vi "Configure Protocol Settings.vi"(8 "error in":errorcluster, 11 "Protocol settings":T1={"Protocol capture resource name"="", "Data line"=0, "Channel"=0, "Clock rate"=12288000, "Number of words"=19200, "Sensitivity"=0.34762, "Frame Sync Edge for Channel 0"=enum."Falling", "Channel Count Per Frame"=2, "Channel Length"=32, "Bit Depth"=24, "Channel 0 Offset"=1, "Endianness"=enum."MSB First", "Data Justification"=enum."Left Justified", "Frame Length"=64, "Frame Sync Pulse Width"=32, "Bit Clock Edge  Sync"=enum."Falling"}) -> (0 "error out":errorcluster, 3 "PDM task":T2)   [LabVIEW 2021]
uses:
  <vilib>/PDM Acquisition Toolkit/host/Classes/Tasks/PCM Input/Controls/DVR PCM Input Task.ctl
  <vilib>/PDM Acquisition Toolkit/host/Classes/Tasks/PCM Input/PCM Input Task.lvclass
  controls/Protocol settings.ctl
  <vilib>/PDM Acquisition Toolkit/host/Classes/Tasks/PDM Tasks/Controls/Acquisition Mode.ctl
  <vilib>/PDM Acquisition Toolkit/host/Classes/Session/Controls/Logic Levels.ctl
  <vilib>/PDM Acquisition Toolkit/shared/controls/PCM Data Format Configuration.ctl
  <vilib>/PDM Acquisition Toolkit/shared/controls/Digital Edge.ctl
  <vilib>/PDM Acquisition Toolkit/shared/controls/PCM Bit Endianness.ctl
  <vilib>/PDM Acquisition Toolkit/shared/controls/PCM Data Justification.ctl
  <vilib>/PDM Acquisition Toolkit/shared/controls/PCM Frame Sync Control.ctl
  <vilib>/PDM Acquisition Toolkit/host/API/Public/Create Tasks/Create PCM Input Task.vi
  <vilib>/PDM Acquisition Toolkit/host/API/Public/Configure/Timing/Configure Timing - PCM Input Slave.vi
  <vilib>/PDM Acquisition Toolkit/host/API/Public/Configure/PDM Channel/Configure Microphone Sensitivity FSPA - PCM Input Task.vi
  <vilib>/PDM Acquisition Toolkit/host/Classes/Tasks/PDM Tasks/PDM Task.lvclass
  <vilib>/PDM Acquisition Toolkit/host/Classes/Session/DecoderSession.lvclass
  <vilib>/PDM Acquisition Toolkit/host/API/PDM Acquisition Toolkit.lvlib
  <vilib>/PDM Acquisition Toolkit/shared/PDM Shared.lvlib
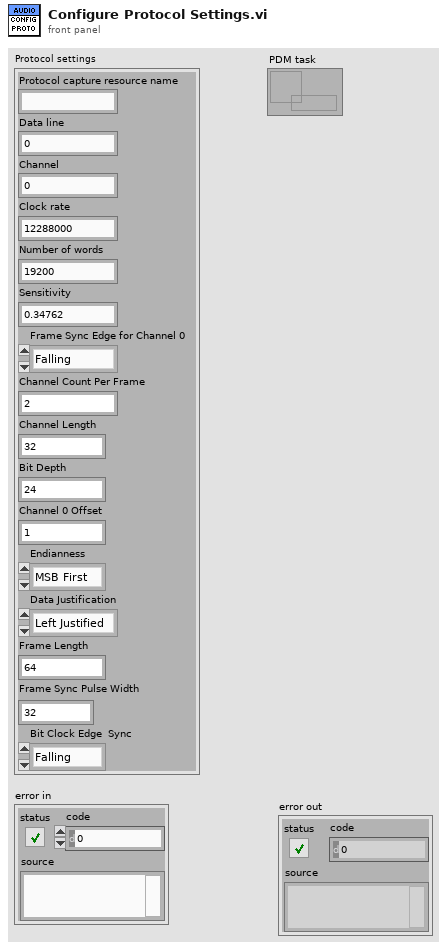
[diagram p1: front panel]
types:
  T1 = typedef "Protocol settings.ctl" = cluster{"Protocol capture resource name":string, "Data line":u16, "Channel":u32, "Clock rate":u32, "Number of words":i32, "Sensitivity":dbl, "Frame Sync Edge for Channel 0":enum16{"Rising", "Falling"}, "Channel Count Per Frame":u8, "Channel Length":u16, "Bit Depth":u8, "Channel 0 Offset":u16, "Endianness":enum16{"MSB First", "LSB First"}, "Data Justification":enum16{"Left Justified", "Right Justified"}, "Frame Length":u16, "Frame Sync Pulse Width":u16, "Bit Clock Edge  Sync":enum8{"Rising", "Falling"}}
  T2 = typedef "PDM Acquisition Class Library.lvlib/PCM Input Task.lvclass/DVR PCM Input Task.ctl" = refnum<data-value>
  T3 = typedef "PDM Shared.lvlib/PCM Frame Sync Control.ctl" = cluster{"Frame Length":u16, "Frame Sync Pulse Width":u16, "Bit Clock Edge  Sync":T4}
  T4 = typedef "PDM Shared.lvlib/Digital Edge.ctl" = enum8{"Rising", "Falling"}
  T5 = typedef "PDM Shared.lvlib/PCM Data Format Configuration.ctl" = cluster{"Frame Sync Edge for Channel 0":T4, "Channel Count Per Frame":u8, "Channel Length":u16, "Bit Depth":u8, "Channel 0 Offset":u16, "Endianness":T6, "Data Justification":T7}
  T6 = typedef "PDM Shared.lvlib/PCM Bit Endianness.ctl" = enum16{"MSB First", "LSB First"}
  T7 = typedef "PDM Shared.lvlib/PCM Data Justification.ctl" = enum16{"Left Justified", "Right Justified"}
  T8 = typedef "PDM Acquisition Class Library.lvlib/DecoderSession.lvclass/Logic Levels.ctl" = enum16{"3.3 V", "1.8 V", "1.2 V"}
  T9 = typedef "PDM Acquisition Class Library.lvlib/PDM Task.lvclass/Acquisition Mode.ctl" = enum16{"Finite", "Continuous"}
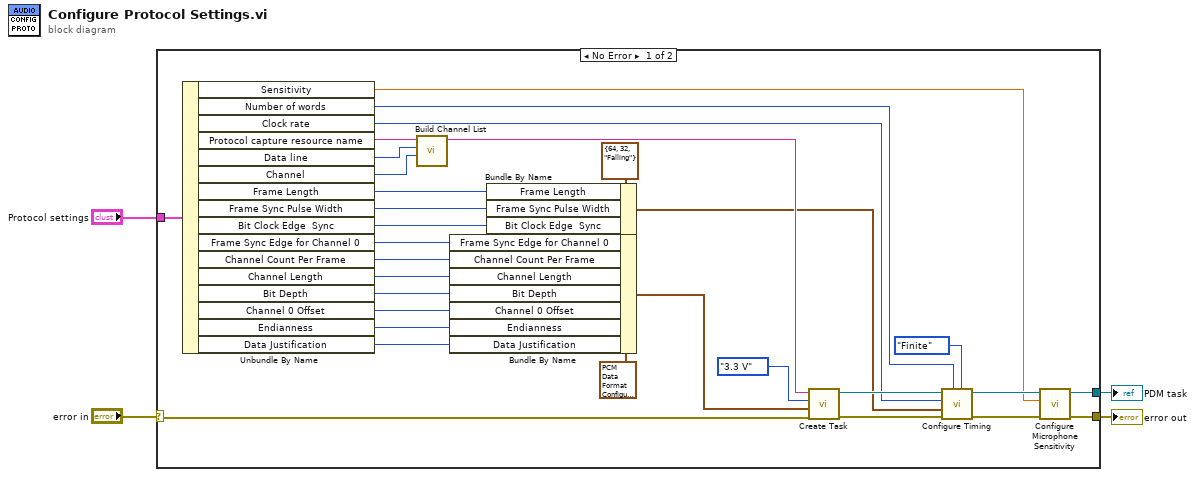
[diagram p0: block diagram]
diagram:
  n1 = case shown="No Error" "error in" {
    selector: "error in" -> [w25 w36]
    tunnel: [w15 w36] -> w2
    tunnel: [w31 _] -> w3
    tunnel: "Protocol settings" -> [w24 _]
    frame No Error {
      n2 = Unbundle By Name(w24) -> ("Sensitivity"=w28:dbl, "Number of words"=w27:i32, "Clock rate"=w26:u32, "Protocol capture resource name"=w23:string, "Data line"=w22:u16, "Channel"=w21:u32, "Frame Length"=w7:u16, "Frame Sync Pulse Width"=w6:u16, "Bit Clock Edge  Sync"=w5:enum8{"Rising", "Falling"}, "Frame Sync Edge for Channel 0"=w10:enum16{"Rising", "Falling"}, "Channel Count Per Frame"=w8:u8, "Channel Length"=w9:u16, "Bit Depth"=w14:u8, "Channel 0 Offset"=w13:u16, "Endianness"=w12:enum16{"MSB First", "LSB First"}, "Data Justification"=w11:enum16{"Left Justified", "Right Justified"})
      n3 = call "Build Channel List.vi"("Channel"=w21, "Data line"=w22, "Protocol capture resource name"=w23) -> ("String"=w20:string)  [unwired: 8 in]
      n4 = Bundle By Name(cluster=T5 {"Frame Sync Edge for Channel 0"=enum."Falling", "Channel Count Per Frame"=2, "Channel Length"=32, "Bit Depth"=24, "Channel 0 Offset"=1, "Endianness"=enum."MSB First", "Data Justification"=enum."Left Justified"} ("PCM data configuration"), "Frame Sync Edge for Channel 0"=w10, "Channel Count Per Frame"=w8, "Channel Length"=w9, "Bit Depth"=w14, "Channel 0 Offset"=w13, "Endianness"=w12, "Data Justification"=w11) -> (w18:T5)
      n5 = Bundle By Name(cluster=T3 {"Frame Length"=64, "Frame Sync Pulse Width"=32, "Bit Clock Edge  Sync"=enum."Falling"} ("Frame Sync Clock Control"), "Frame Length"=w7, "Frame Sync Pulse Width"=w6, "Bit Clock Edge  Sync"=w5) -> (w16:T3)
      n6 = call-poly <vilib>:"Create Task.vi"("error in"=w25, "PCM data configuration"=w18, "logic level"=Logic_Levels."3.3 V", "channel list"=w20) -> ("error out"=w34:errorcluster, "PCM input task out"=w35:T2)  [unwired: 6 in]
      n7 = call-poly <vilib>:"Configure Timing.vi"("acquisition mode"=Acquisition_Mode."Finite", "Frame Sync Clock Control"=w16, "number of words per channel"=w27, "error in"=w34, "Bit Clock rate"=w26, "PCM input task in"=w35) -> ("error out"=w29:errorcluster, "PCM input task out"=w30:T2)  [unwired: 4 in]
      n8 = call-poly <vilib>:"Configure Microphone Sensitivity.vi"("error in"=w29, "microphone sensitivity (FS/Pa)"=w28, "PCM input task in"=w30) -> ("error out"=w15:errorcluster, "PCM input task out"=w31:T2)  [unwired: 7 in]
    }
    frame Error {
    }
  }
  "PDM task" <- w3
  "error out" <- w2
